vi "Read All.vi"(4 "TypeMap in":refnum<class "TypeMap.lvclass">, 5 "Options":T1, 6 "commandTimeout":i32=-1, 7 "Limit":i64, 8 "error in (no error)":errorcluster, 9 "Where":string[](array[string]), 10 "Object":refnum<class>, 11 "SqlMapper in":refnum<class "SqlMapper.lvclass">) -> (0 "error out":errorcluster, 2 "Query Results":refnum<class>[](array[class]), 3 "SqlMapper out":refnum<class "SqlMapper.lvclass">)   [LabVIEW 2020, in "ORM_API.lvlib"]
uses:
  ORM_API.lvlib
  <vilib>/Viviota/shared/ORM.lvlibp/ORM/TypeMap/TypeMap.lvclass
  <vilib>/Viviota/shared/ORM.lvlibp/ORM/SqlMapper/SqlMapper.lvclass
  <userlib>/_OpenG.lib/lvdata/lvdata.llb/LVOOP Is Default Value__ogtk.vi
  <vilib>/Viviota/shared/ORM.lvlibp/ORM/TypeMap/Read TypeMap.vi
  <vilib>/Viviota/shared/ORM.lvlibp/ORM/Query Result/Next.vi
  <vilib>/Viviota/shared/ORM.lvlibp/ORM/TypeMap/ToLabVIEW_Wrap.vi
  <vilib>/Viviota/shared/ORM.lvlibp/ORM/Query Result/Query Result.lvclass
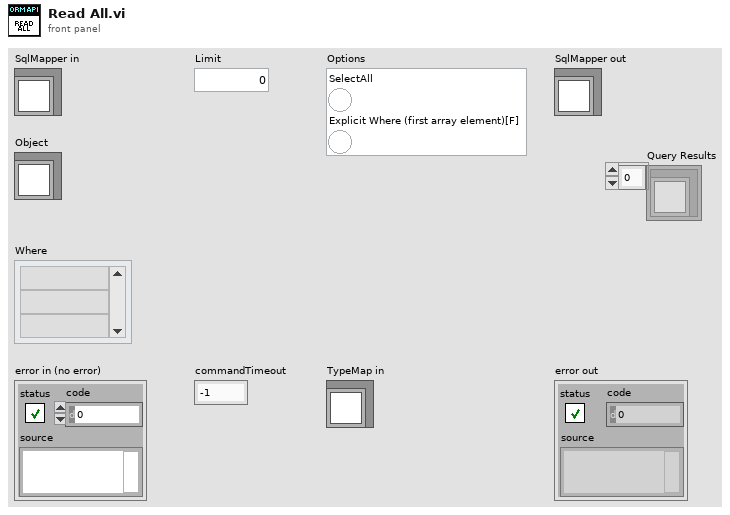
[diagram p1: front panel]
types:
  T1 = cluster{"SelectAll":bool, "Explicit Where (first array element)[F]":bool}
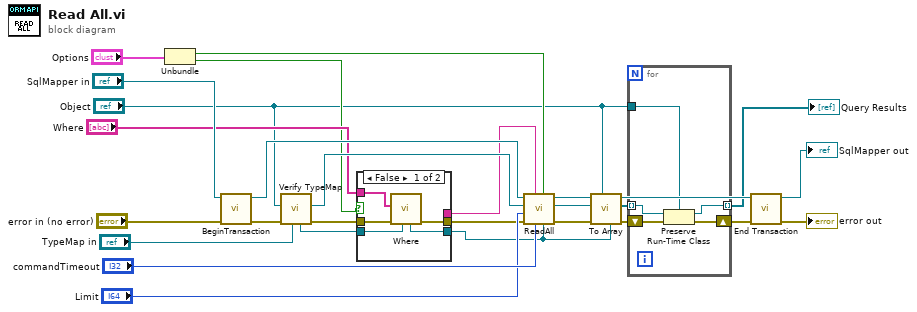
[diagram p0: block diagram]
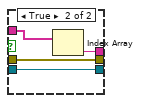
[diagram p2: hidden frame]
diagram:
  n1 = Unbundle("Options") -> ("SelectAll"=w6:bool, "Explicit Where (first array element)[F]"=w7:bool)
  n2 = call-dynamic "BeginTransaction.vi"("error in (no error)"="error in (no error)", "SqlMapper in"="SqlMapper in") -> ("error out"=w28:errorcluster, "SqlMapper out"=w24:refnum<class "SqlMapper.lvclass">)  [unwired: 8 in]
  n3 = call "Verify TypeMap.vi"("TypeMap in"="TypeMap in", "error in (no error)"=w28, "Type in"="Object") -> ("error out"=w12:errorcluster, "Type out"=w20:refnum<class>, "TypeMap out"=w11:refnum<class "TypeMap.lvclass">)  [unwired: 6 in]
  n4 = case shown="False" w7 {
    tunnel: w12 -> [w33 w36]
    tunnel: [w32 w36] -> w13
    tunnel: w11 -> [w31 w37]
    tunnel: [w30 w37] -> w10
    tunnel: [_ w35] -> w9
    tunnel: "Where" -> [w29 w34]
    frame False {
      n5 = call <vilib>:"Where.vi"("TypeMap in"=w31, "error in (no error)"=w33, "Where in"=w29) -> ("error out"=w32:errorcluster, "TypeMap out"=w30:refnum<class "TypeMap.lvclass">)  [unwired: 7 in]
    }
    frame True {
      n6 = Index Array(array=w34) -> (element=w35:string)  [unwired: 1 in]
    }
  }
  n7 = call-dynamic "ReadAll.vi"("TypeMap in"=w10, "Select *"=w6, "commandTimeout"="commandTimeout", "Where"=w9, "error in (no error)"=w13, "Limit"="Limit", "object in"=w20, "SqlMapper in"=w24) -> ("error out"=w18:errorcluster, "Query Result out"=w17:refnum<class "Query Result.lvclass">, "SqlMapper out"=w16:refnum<class "SqlMapper.lvclass">)  [unwired: 1 in]
  n8 = call "To Array.vi"("TypeMap"=w10, "Type"="Object", "error in (no error)"=w18, "Query Result in"=w17, "SqlMapper in"=w16) -> ("error out"=w3:errorcluster, "Array"=w5:refnum<class>[], "SqlMapper out"=w15:refnum<class "SqlMapper.lvclass">)  [unwired: 4 in]
  n9 = for {
    tunnel: w5 -> [w40] mode=indexing
    tunnel: [w39] -> w2 mode=indexing
    tunnel: "Object" -> [w38]
    shift-right: [w41] -> w4
    shift-left: w3 -> [w42]
    n10 = Preserve Run-Time Class(object in=w40, error in=w42, 2:w38) -> (object out=w39:refnum<class>, error out=w41:errorcluster)
  }
  "Query Results" <- w2
  n11 = call <vilib>:"End Transaction.vi"("error in (no error)"=w4, "SqlMapper in"=w15) -> ("error out"=→"error out":errorcluster, "SqlMapper out"=→"SqlMapper out":refnum<class "SqlMapper.lvclass">)  [unwired: 8 in]
